vi "Read Attitude Msg.vi"(11 "TCP  Refnum In":refnum<k5>) -> (1 "MT_DATA":dbl[](array[numeric]), 3 "TCP Refnum Out":refnum<k5>, 4 "Omega Estimated":dbl[](array[numeric]), 5 "Theta Estimated":dbl[](array[numeric]), 6 "Omega Measured":dbl[](array[numeric]), 7 "Theta Measured":dbl[](array[numeric]))   [LabVIEW 2014]
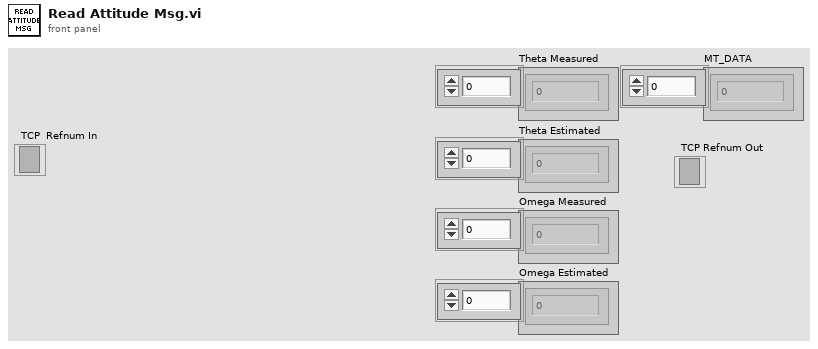
[diagram p1: front panel]
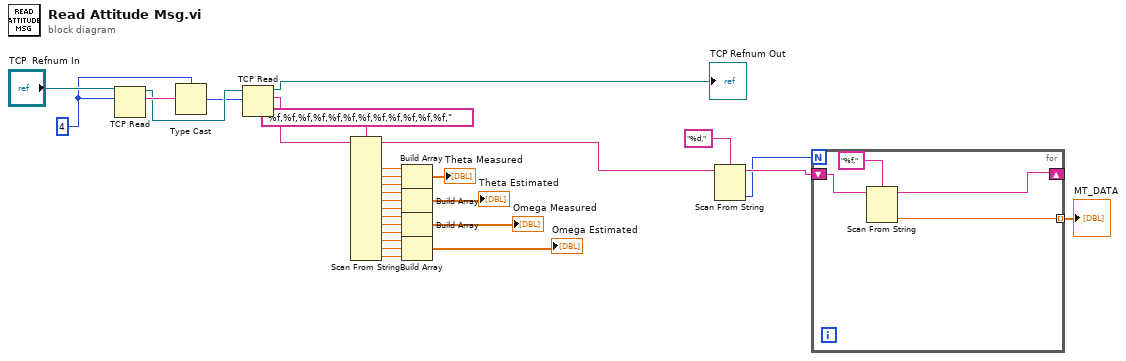
[diagram p0: block diagram]
diagram:
  w27 = 4
  n1 = TCP Read(connection ID="TCP  Refnum In", bytes to read=w27) -> (connection ID out=w26:refnum<k5>, data out=w28:string)  [unwired: 3 in, 1 out]
  n2 = Type Cast(type=w27, x=w28) -> (*(type *) &x=w25:i32)
  n3 = TCP Read(connection ID=w26, bytes to read=w25) -> (connection ID out=→"TCP Refnum Out":refnum<k5>, data out=w23:string)  [unwired: 3 in, 1 out]
  n4 = Scan From String(format string="%f,%f,%f,%f,%f,%f,%f,%f,%f,%f,%f,%f,", input string=w23) -> (remaining string=w5:string, output 1=w21:dbl, output 2=w20:dbl, output 3=w19:dbl, output 4=w18:dbl, output 5=w17:dbl, output 6=w16:dbl, output 7=w15:dbl, output 8=w14:dbl, output 9=w13:dbl, output 10=w12:dbl, output 11=w11:dbl, output 12=w10:dbl)  [unwired: 14 in, 2 out]
  n5 = Build Array(w21, w20, w19) -> (→"Theta Measured":dbl[])
  n6 = Build Array(w18, w17, w16) -> (→"Theta Estimated":dbl[])
  n7 = Build Array(w15, w14, w13) -> (→"Omega Measured":dbl[])
  n8 = Build Array(w12, w11, w10) -> (→"Omega Estimated":dbl[])
  n9 = Scan From String(format string="%d,", input string=w5) -> (remaining string=w3:string, output 1=w2:i32)  [unwired: 3 in, 2 out]
  n10 = for {
    N: w2 -> [_]
    shift-right: [w32] -> _
    shift-left: w3 -> [w33]
    tunnel: [w31] -> w1 mode=indexing
    n11 = Scan From String(format string="%f,", input string=w33) -> (remaining string=w32:string, output 1=w31:dbl)  [unwired: 3 in, 2 out]
  }
  "MT_DATA" <- w1
